vi "Set Temperature Range.vi"(8 "error in (no error)":errorcluster, 9 "Min":dbl, 10 "Max":dbl, 11 "Optris PI in":refnum<class "Optris PI.lvclass">) -> (0 "error out":errorcluster, 3 "Optris PI out":refnum<class "Optris PI.lvclass">)   [LabVIEW 2018, in "Optris PI.lvlib" / "Optris PI.lvclass"]
uses:
  Optris PI.lvclass
  <instrlib>/Optris PI/libirimager_direct_binding.lvlib
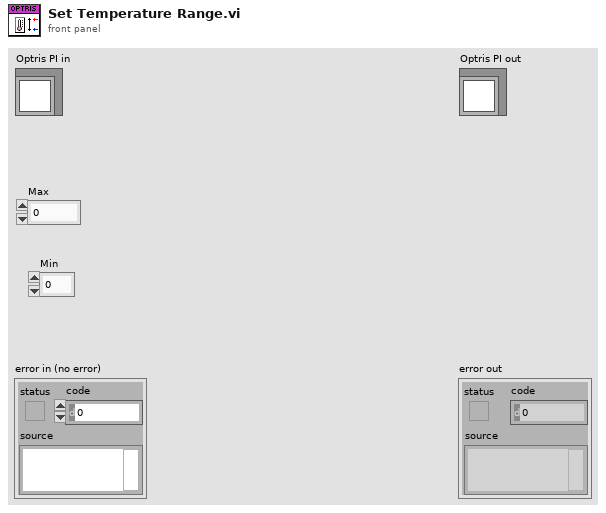
[diagram p1: front panel]
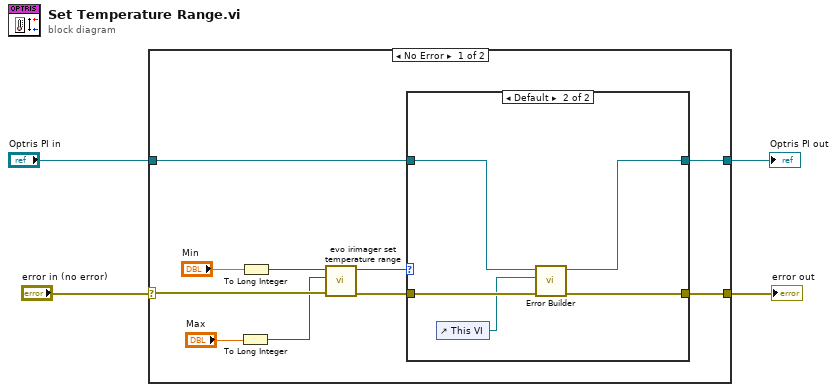
[diagram p0: block diagram]
diagram:
  n1 = case shown="No Error" "error in (no error)" {
    selector: "error in (no error)" -> [w14 w22]
    tunnel: [w8 w23] -> w3
    tunnel: "Optris PI in" -> [w7 w23]
    tunnel: [w5 w22] -> w1
    frame No Error {
      n2 = To Long Integer(number="Max") -> (32bit integer=w12:i32)
      n3 = To Long Integer(number="Min") -> (32bit integer=w10:i32)
      n4 = call <instrlib>:"evo irimager set temperature range.vi"("error in (no error)"=w14, "t_max"=w12, "t_min"=w10) -> ("error out"=w6:errorcluster, "function return"=w9:i32)  [unwired: 7 in]
      n5 = case shown="Default" w9 {
        tunnel: [w16 w18] -> w8
        tunnel: w7 -> [w16 w19]
        tunnel: w6 -> [w15 w21]
        tunnel: [w15 w20] -> w5
        frame 0 {
        }
        frame Default {
          n6 = control-ref of="This VI"() -> (w17:refnum<vi>)
          n7 = call "Error Builder.vi"("error in (no error)"=w21, "This VI"=w17, "Optris PI in"=w19) -> ("Error out"=w20:errorcluster, "Optris PI out"=w18:refnum<class "Optris PI.lvclass">)  [unwired: 7 in]
        }
      }
    }
    frame Error {
    }
  }
  "error out" <- w1
  "Optris PI out" <- w3
